vi "BIMS_Assembler.vi"() -> ()   [LabVIEW 2010]
doc: "This program is currently beta software. It is designed to address the data requirements defined primarily by the DHB Ballistic Test Report.\n\nThe general operation of this program is based on the Ballistics Version 2005 application developed internally by DuPont as a research tool for the Spruance Plant Ballistics Lab in Richmond, VA.\n\nPlease note that the original trigger control logic was modified and no longer depends on a safety interlock system to enable operation of a ballistic test.\n\nDuPont makes no warranties and assumes no liabilities in connection with any use of this program."
uses:
  Collector State.ctl
  <vilib>/registry/registry.llb/Registry RtKey.ctl
  BIMS_Collector Globals.vi
panel:
  out "Loading":u16(ring)
  in  "runtimeMenusVisible":bool=TRUE
  in  "diagPageVisible":bool
  in  "RESET All":bool
  out "ConfigName":string
  out "TimeNow":string
  in  "EXIT":bool
  in  "mainTabCntrl":enum32{"Setup", "System"}(tab)
  in  "Sample SubTabCntrl":T1(tab)
  in  "NewProject":bool
  in  "# of Panels":dbl
  in  "SampleID":string caption="Sample ID"
  in  "SampleDimensions":u16(ring) caption="Dimensions" items=["", "15 x 15", "12 x 12", "10.25 x 11.75", "15 x 16", "26 x 26", "8.5 x 11", "12 x 15", "16 x 16", "18 x 18", "20 x 16", "15 x 18", "24 x 24", "13 x 13", "7.5 x 7.5", "VEST PANEL", "CHEST PLATE", "HELMET", "NOT APPLICABLE"]
  in  "ModelMfrs":u16(ring) caption="Manufacturer" items=["DuPont Experimental", "Clark Schwebel", "Industriales Textiles", "Maydown", "Second Chance Body Armor", "Point Blank-Marine Interceptor", "Safari Land", "American Body Armor", "Europe", "Force One", "Textile Filter", "Hexcel Schwebel", "BGF", "M.C. GILL", "COLUMBIA", "Britax HEATH TECN", "ARLON", "TEX TECH INC.", "TELAIR", "CADDIN BODY ARMOR", "GEPCO", "3 TEX", "PACA BODY ARMOR", "VON ROL ISOLA", "SIOUX MANUFACTURING", "APEJ-TAIWAN", "FLOPPY BODY ARMOR", "UNICOR", "n/a", "Point Blank", "Diamond Back", "Other"]
  in  "SampleTypes":u16(ring) caption="Sample Type" items=["", "Fabric", "Hard", "Helmet", "Vest", "Paper"]
  in  "Submitters":u16(ring) caption="Submitter" items=["", "Aldo Tavarez", "James Singletary", "Jeff Hanks", "Karl Chang", "Minshon Chiou", "Other", "Navin Tejani", "Pat Fitzgerald", "Ron Egres", "Bryce VanArsdalen", "Kevin Mulcahy"]
  out "ProjectID":string caption="Project ID"
  in  "BackLayers":i32 caption="# of Layers" min=0 max=99 step=5
  in  "FrontLayers":i32 caption="# of Layers" min=0 max=99 step=5
  in  "BackLayer":u16(ring) caption="Back Layer" items=["", "n/a", "CORDURA 500d"]
  in  "FrontLayer":u16(ring) caption="Front Layer" items=["", "n/a", "CORDURA 1000d"]
  out "totalNumLayers":i32 caption="Total # of Layers" min=0 max=100 step=5
  out "totalBAW":sgl caption="Total BAW (psf)" format="%.2f"
  in  "LayerTabControl":enum32{"1", "2", "3", "4", "5", "6"}(tab) caption="Inner Layers"
  out "fab1_totalWt":sgl caption="Fab1 Wt" min=0 max=99 step=5 format="%.2f"
  out "SampleAttribs_1":T2 caption="fabricAttribs_1"
  in  "Layer_1":T3={"plyNum"=0, "LotNum"="n/a", "RollNum"="n/a"} caption="Fabric #1" {"plyNum" min=0 max=99 step=5}
  in  "SampleStyle_1":u16(ring)
  in  "Mfr_1":u16(ring) caption="vendor" items=["", "Barrday", "DSM", "DuPont AFS", "Dyneema", "Honeywell", "JPS", "TexTech"]
  in  "layerStitch_1":u16(ring) caption="Stitch" items=["", "1-inch quilt", "2-inch quilt", "Corner Bartack", "Corners", "Custom (Panel)", "Custom (Vest)", "Diamond", "Edge", "n/a", "Normal"]
  out "fab2_totalWt":sgl caption="Fab2 Wt" min=0 max=99 step=5 format="%.2f"
  out "SampleAttribs_2":T2 caption="fabricAttribs_2"
  in  "Layer_2":T3={"plyNum"=0, "LotNum"="n/a", "RollNum"="n/a"} caption="Fabric #2" {"plyNum" min=0 max=99 step=5}
  in  "SampleStyle_2":u16(ring)
  in  "Mfr_2":u16(ring) caption="vendor" items=["", "Barrday", "DSM", "DuPont AFS", "Dyneema", "Honeywell", "JPS", "TexTech"]
  in  "layerStitch_2":u16(ring) caption="Stitch" items=["", "1-inch quilt", "2-inch quilt", "Corner Bartack", "Corners", "Custom (Panel)", "Custom (Vest)", "Diamond", "Edge", "n/a", "Normal"]
  out "fab3_totalWt":sgl caption="Fab3 Wt" min=0 max=99 step=5 format="%.2f"
  out "SampleAttribs_3":T2 caption="fabricAttribs_3"
  in  "Layer_3":T3={"plyNum"=0, "LotNum"="n/a", "RollNum"="n/a"} caption="Fabric #3" {"plyNum" min=0 max=99 step=5}
  in  "SampleStyle_3":u16(ring)
  in  "Mfr_3":u16(ring) caption="vendor" items=["", "Barrday", "DSM", "DuPont AFS", "Dyneema", "Honeywell", "JPS", "TexTech"]
  in  "layerStitch_3":u16(ring) caption="Stitch" items=["", "1-inch quilt", "2-inch quilt", "Corner Bartack", "Corners", "Custom (Panel)", "Custom (Vest)", "Diamond", "Edge", "n/a", "Normal"]
  out "fab4_totalWt":sgl caption="Fab4 Wt" min=0 max=99 step=5 format="%.2f"
  out "SampleAttribs_4":T2 caption="fabricAttribs_4"
  in  "Layer_4":T3={"plyNum"=0, "LotNum"="n/a", "RollNum"="n/a"} caption="Fabric #4" {"plyNum" min=0 max=99 step=5}
  in  "SampleStyle_4":u16(ring)
  in  "Mfr_4":u16(ring) caption="vendor" items=["", "Barrday", "DSM", "DuPont AFS", "Dyneema", "Honeywell", "JPS", "TexTech"]
  in  "layerStitch_4":u16(ring) caption="Stitch" items=["", "1-inch quilt", "2-inch quilt", "Corner Bartack", "Corners", "Custom (Panel)", "Custom (Vest)", "Diamond", "Edge", "n/a", "Normal"]
  out "fab5_totalWt":sgl caption="Fab5 Wt" min=0 max=99 step=5 format="%.2f"
  out "SampleAttribs_5":T2 caption="fabricAttribs_5"
  in  "Layer_5":T3={"plyNum"=0, "LotNum"="n/a", "RollNum"="n/a"} caption="Fabric #5" {"plyNum" min=0 max=99 step=5}
  in  "SampleStyle_5":u16(ring)
  in  "Mfr_5":u16(ring) caption="vendor" items=["", "Barrday", "DSM", "DuPont AFS", "Dyneema", "Honeywell", "JPS", "TexTech"]
  in  "layerStitch_5":u16(ring) caption="Stitch" items=["", "1-inch quilt", "2-inch quilt", "Corner Bartack", "Corners", "Custom (Panel)", "Custom (Vest)", "Diamond", "Edge", "n/a", "Normal"]
  out "fab6_totalWt":sgl caption="Fab6 Wt" min=0 max=99 step=5 format="%.2f"
  out "SampleAttribs_6":T2 caption="fabricAttribs_6"
  in  "Layer_6":T3={"plyNum"=0, "LotNum"="n/a", "RollNum"="n/a"} caption="Fabric #6" {"plyNum" min=0 max=99 step=5}
  in  "SampleStyle_6":u16(ring)
  in  "Mfr_6":u16(ring) caption="vendor" items=["", "Barrday", "DSM", "DuPont AFS", "Dyneema", "Honeywell", "JPS", "TexTech"]
  in  "layerStitch_6":u16(ring) caption="Stitch" items=["", "1-inch quilt", "2-inch quilt", "Corner Bartack", "Corners", "Custom (Panel)", "Custom (Vest)", "Diamond", "Edge", "n/a", "Normal"]
  in  "SampleCoverings":u16(ring) caption="Sample Covering" items=["None", "RipStop", "Plastic bag", "Other"]
  in  "Assemblers":u16(ring) caption="Technician" items=["", "Not Known", "none", "Ron Egres", "Bryce VanArsdalen", "Mary Revels", "Matthew Street", "Patty Whitlow", "Tom Boyer"]
  in  "Thickness":dbl caption="Thickness (in)" format="%.3f"
  in  "totalSampleWt":sgl caption="Total Weight (lbs)" format="%.3f"
  in  "Comments":string caption="Remarks (optional):"
  in  "TestConditions":u16(ring) caption="Sample Condition" items=["", "Dry", "Wet", "Hot 160 DEG. F", "Cold", "Weapon Lubricant", "Motor Oil", "Conditioned", "Accelerated Aging"]
  in  "aboutTabCntrl":enum32{"About ", "Internal Use"}(tab)
  in  "RefreshMetadata":bool
  in  "PublishNewRecords":bool
  in  "clearErrors":bool
  in  "Server":string="esvrs11"
  in  "Site":string="ICE1"
  in  "processShots":bool
  in  "line direction map":i32=1792 format="%.0b"
  in  "old threat":u16
  in  "Areal Density":dbl format="%.2f"
  in  "Areal density text":string
  in  "Fabric Description":string caption="Fabric Desc"
  out "configPath":path=path "P:/Private/My Projects/AFS/BIMS/2008/BIMS_Collector.ini" caption="Configuration Path (INI)"
  in  "Threat":u16(ring) caption="Threat (long description)"
  out "massUnits":string="GRAMS" caption="Weight Units"
  out "lengthUnits":string="FOOT" caption="Distance Units"
  in  "SampleDescrip":u16(ring) caption="Misc. Sample Description (legacy)"
  in  "serialNum":string caption="Serial #"
  in  "Models":u16(ring) caption="Model #" items=["n/a"]
  out "SMErr":errorcluster
  out "U/I EvErr":errorcluster
  out "booleanDump":bool
  in  "LayerStitchTypes":u16(ring) caption="Stitch" items=["", "Custom (Vest)", "Corners", "1-inch quilt", "2-inch quilt", "Normal", "Custom (Panel)", "Corner Bartack", "Diamond", "Edge", "n/a"]
  # "Effectively restarts the application from scratch, as if the user pressed the EXIT button and then restarted the application."
  # "Configured for"
  # "Body Side"
  # "Strike Face"
  # "Layer"
  # "Mfr"
  # "Style"
  # "# of Plies"
  # "Lot"
  # "Roll"
  # "Stitch"
  # "Internal ID"
  # "Fiber"
  # "Denier"
  # "Pick"
  # "Weave"
  # "Finish"
  # "oz/yd²"
  # "Asset"
  # "Total Weight"
  # "1"
  # "2"
  # "3"
  # "4"
  # "5"
  # "6"
  # "DuPont Ballistics Information Management System\n\nBIMS\nEnterprise Edition\n\n\nSample Assembler\n\nJanuary 2009"
  # "DuET Measurement System Technologies\nDUCOM 8 695-2330 for technical support\n\nCopyright © 2009 DuPont Company"
  # "Deployment Configuration"
  # "Data items support Point Blank requirements:"
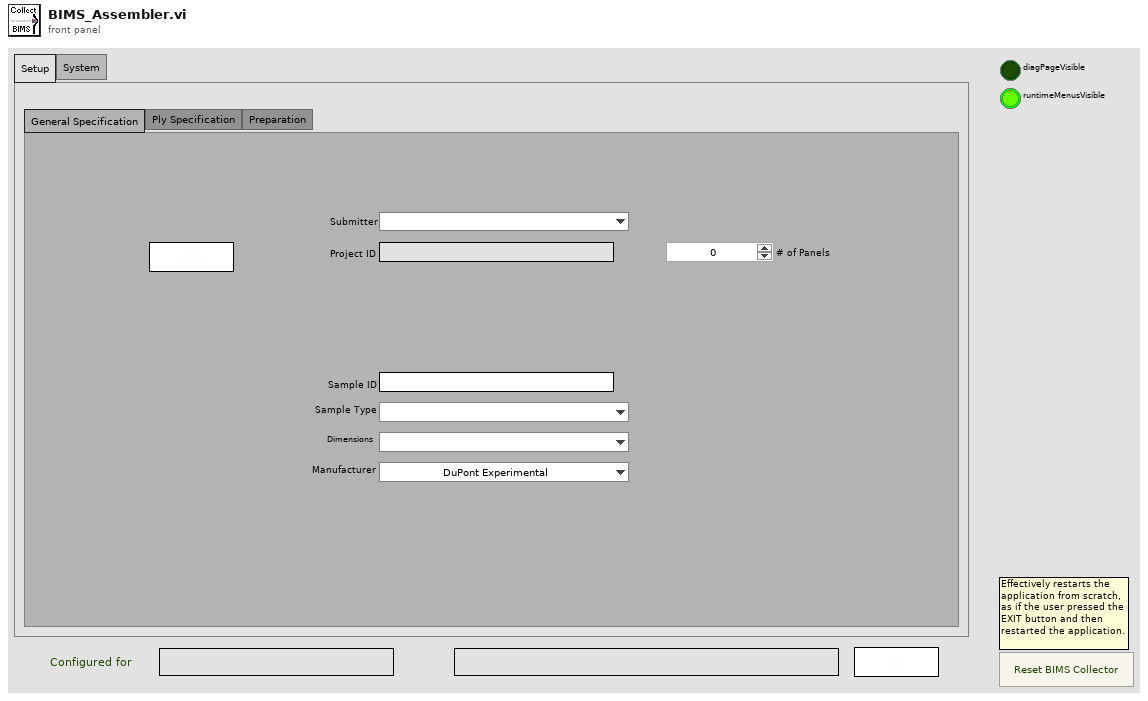
[diagram p1: front panel]
types:
  T1 = enum32{"General Specification", "Ply Specification", "Preparation"}
  T2 = cluster{"Fabric.fiber":string, "Fabric.denier":string, "pick":string, "weave":string, "finish":string, "ozPerYd2":string, "fabricID_DHB":string, "asset":string}
  T3 = cluster{"plyNum":i32, "LotNum":string, "RollNum":string}
  T4 = typedef "Collector State.ctl" = enum16{"POLL", "INITIALIZE", "V50 Report or GET Record", "VsVr Report", "SAVE SHOTS", "ADD SHOT", "CLEAR SHOTS", "NEXT SHOT", "DELETE SHOT", "PROCESS SHOTS", "READY CLOCK", "CHECK DAQ"}
  T5 = enum32{"Page Enabled", "Page Disabled", "Page Disabled & Grayed"}
  T6 = typedef "Registry RtKey.ctl" = enum32{"HKEY_CLASSES_ROOT", "HKEY_CURRENT_USER", "HKEY_LOCAL_MACHINE", "HKEY_USERS", "HKEY_PERFORMANCE_DATA", "HKEY_CURRENT_CONFIG", "HKEY_DYN_DATA"}
  T7 = cluster{"SampleTypes":refnum<vi>, "SampleDescrip":refnum<vi>}
  T8 = enum32{"invalid app kind", "Development System", "Run Time System", "Student Edition", "Embedded LabVIEW", "Evaluation", "Custom"}
  T9 = cluster{"fiber":string, "denier":string, "construction":string, "weave":string, "finish":string, "ozPerYd2":string, "fabricStyle_DHB":string, "yarnMerge":string}
  T10 = cluster{"fiber":string, "denier":string, "pick":string, "weave":string, "finish":string, "ozPerYd2":string, "internal_ID":string, "asset":string}[]
  T11 = cluster{"plyNum":i32, "LotNum":string, "RollNum":string}[]
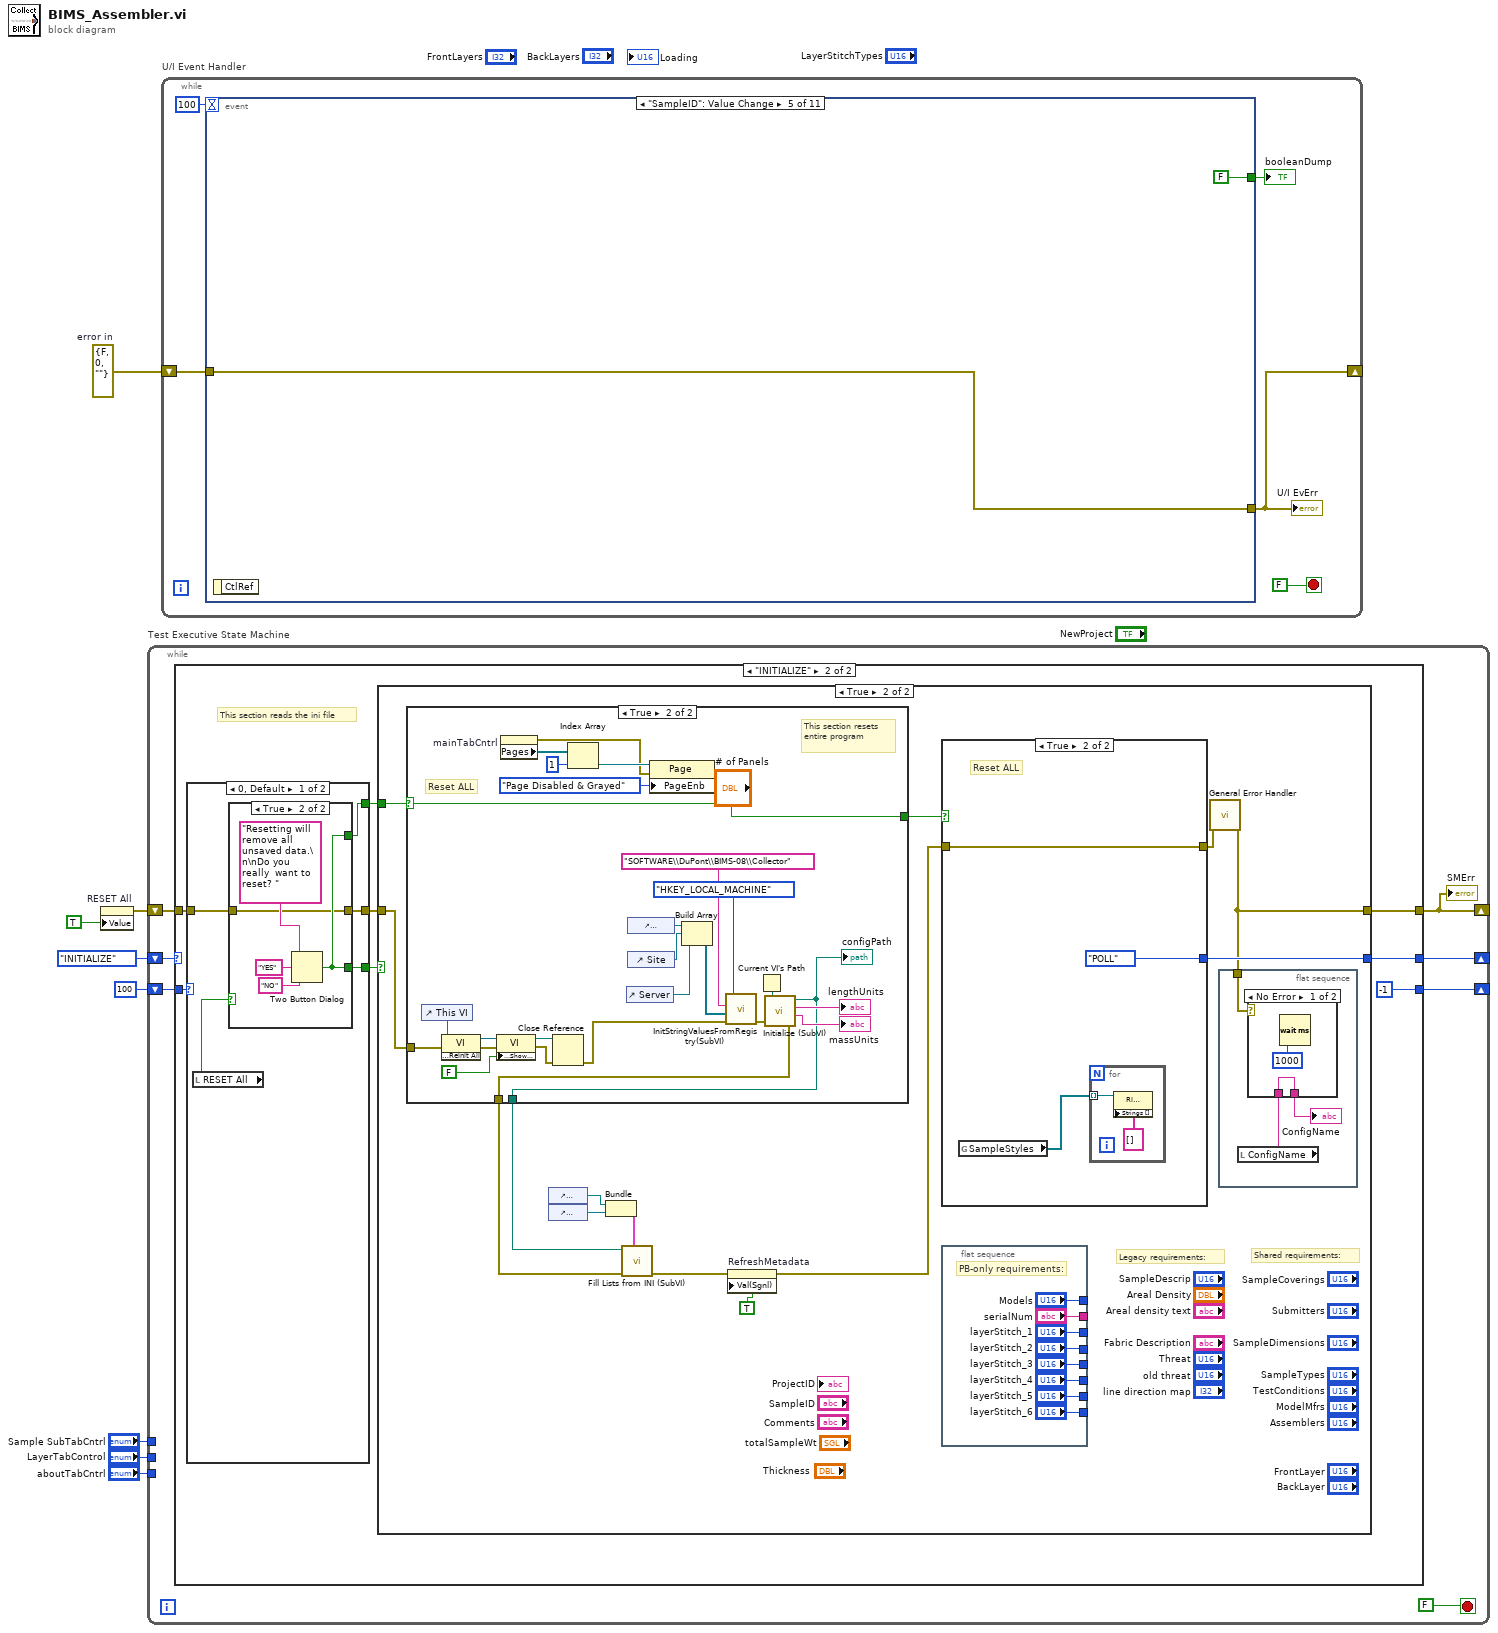
[diagram p0: block diagram]
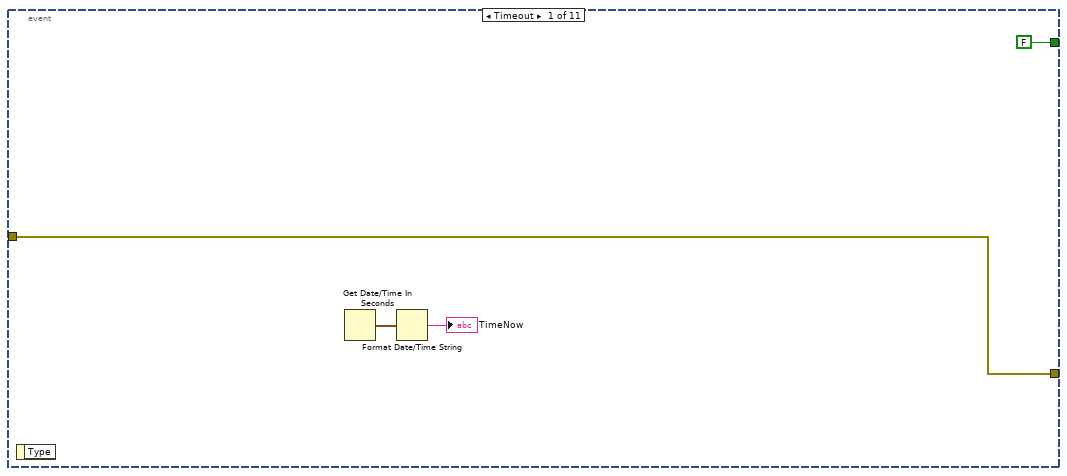
[diagram p2: hidden frame]
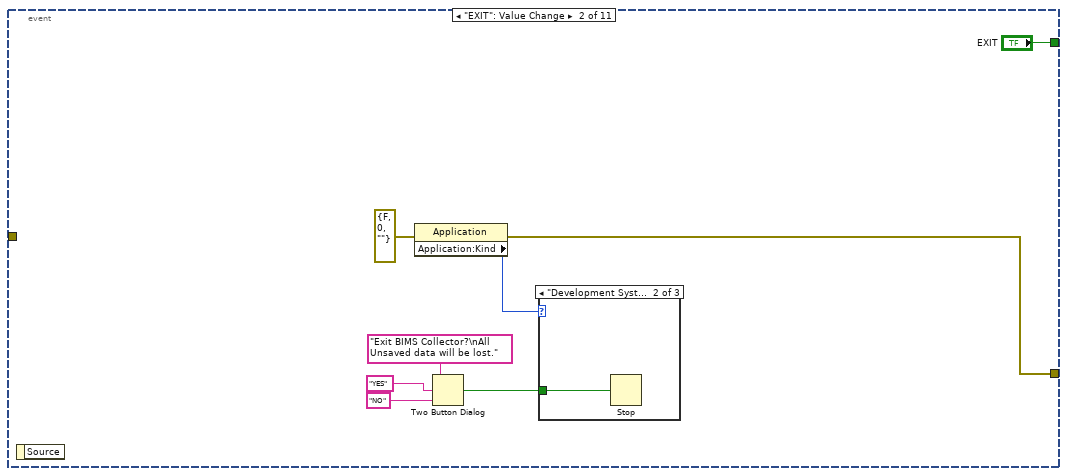
[diagram p3: hidden frame]
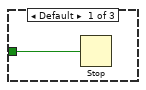
[diagram p4: hidden frame]
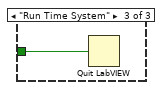
[diagram p5: hidden frame]
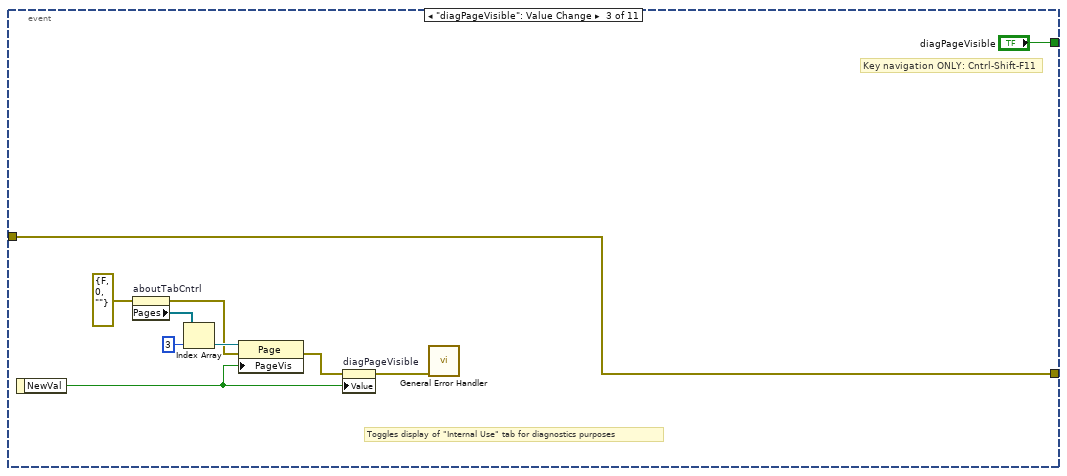
[diagram p6: hidden frame]
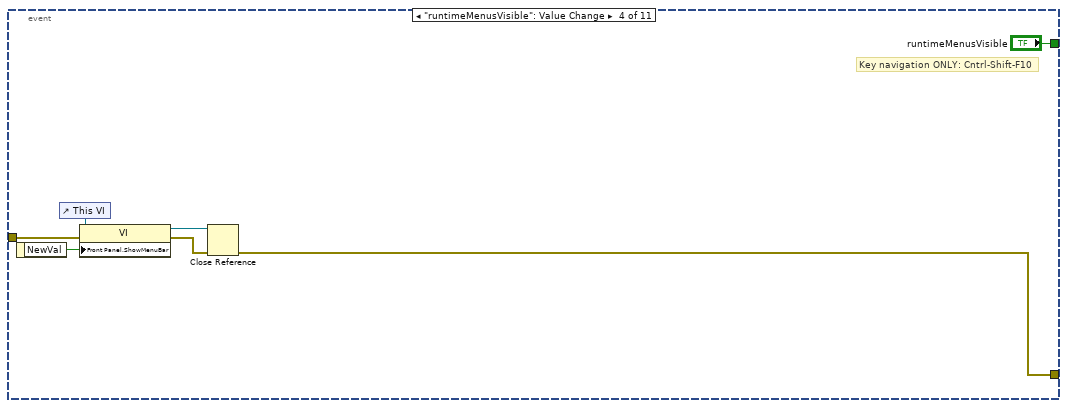
[diagram p7: hidden frame]
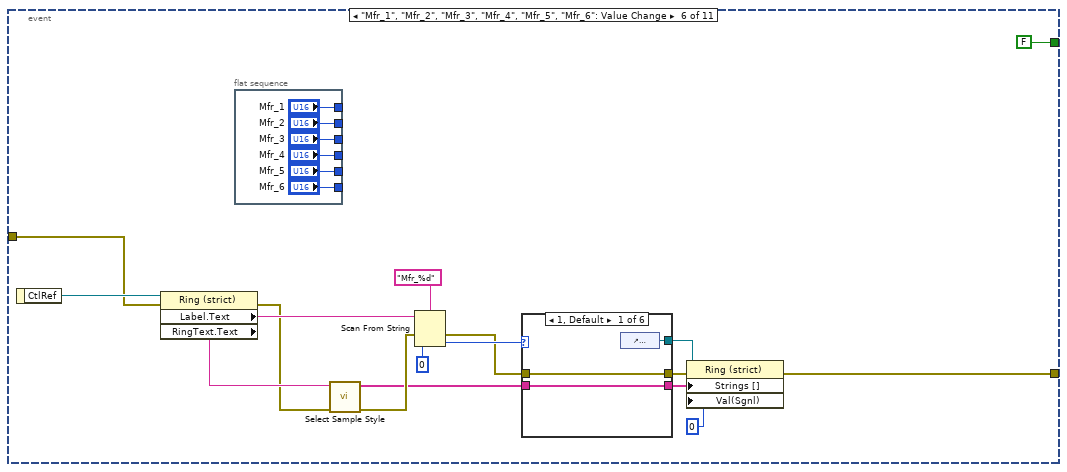
[diagram p8: hidden frame]
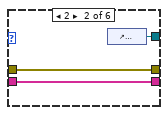
[diagram p9: hidden frame]
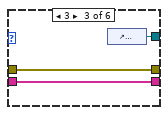
[diagram p10: hidden frame]
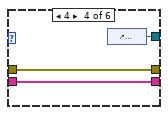
[diagram p11: hidden frame]
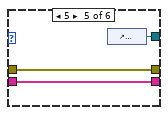
[diagram p12: hidden frame]
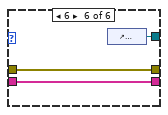
[diagram p13: hidden frame]
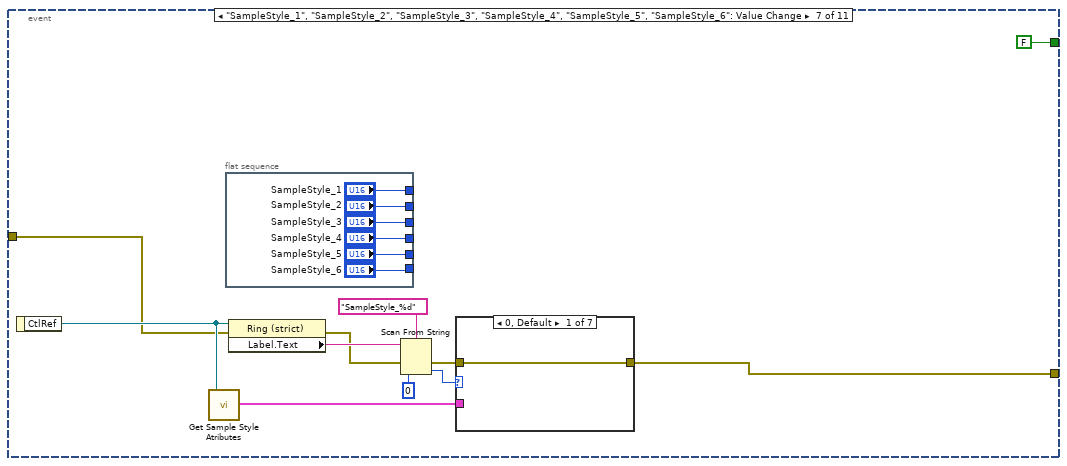
[diagram p14: hidden frame]
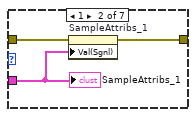
[diagram p15: hidden frame]
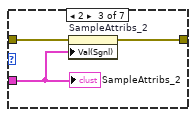
[diagram p16: hidden frame]
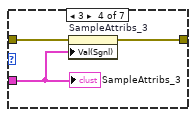
[diagram p17: hidden frame]
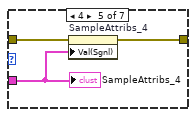
[diagram p18: hidden frame]
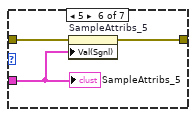
[diagram p19: hidden frame]
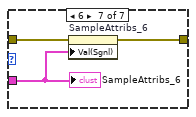
[diagram p20: hidden frame]
diagram:
  w4 = errorcluster {"status"=FALSE, "code"=0, "source"=""}  # error in
  n1 = property on="RESET All" class="Bool (strict)"("Value"=TRUE ("RESET")) -> (error out=w6:errorcluster)  [unwired: 2 in, 1 out]
  n2 = while "Test Executive State Machine" {
    shift-left: 100 -> [w12]
    shift-right: [w13] -> _
    shift-left: Collector_State."INITIALIZE" ("progState") -> [w11]
    shift-right: [w14] -> _
    shift-right: [w9] -> _
    shift-left: w6 -> [w10]
    tunnel: "LayerTabControl" -> [_]
    tunnel: "aboutTabCntrl" -> [_]
    tunnel: "Sample SubTabCntrl" -> [_]
    stop <- FALSE stop-if-true
    n3 = case shown="\"INITIALIZE\"" w11 {
      tunnel: [w22 w33] -> w14
      tunnel: [-1 -1 ("index of element")] -> w13
      tunnel: w12 -> [_ w34]
      tunnel: w10 -> [_ w29]
      tunnel: [w17 w30] -> w9
      frame "POLL", Default {
        w26 = Collector_State."POLL"  # progStateType
        w23 = TRUE  # element
        # "This section checks for any buttons, maintains routine check of the paramters"
        n4 = Build Array("RESET All", "processShots") -> (w24:bool[])
        n5 = Search 1D Array(1D array=w24, element=w23) -> (index of element=w27:i32)  [unwired: 1 out]
        n6 = Increment(x=w27) -> (x+1=w16:i32)
        n7 = local read "SMErr"() -> (w17:errorcluster)
        n8 = To Variant(anything=w16) -> (Variant=w25:variant)
        n9 = Variant To Data(Variant=w25, type=w26) -> (data=w22:T4)  [unwired: 1 in, 1 out]
        n10 = Wait (ms)(milliseconds to wait=u32 200 ("millisecond timer value")) -> ()  [unwired: 1 out]
      }
      frame "INITIALIZE" {
        # "This section reads the ini file"
        n11 = case shown="0, Default" w34 {
          tunnel: [w40 w58] -> w35
          tunnel: [w38 w58] -> w32
          tunnel: w29 -> [w37 w50]
          tunnel: [w36 w50] -> w28
          frame 0, Default {
            n12 = local read "RESET All"() -> (w39:bool)
            n13 = case shown="True" w39 {
              tunnel: [TRUE w47] -> w40
              tunnel: [FALSE w47] -> w38
              tunnel: w37 -> [w41 w44]
              tunnel: [w41 w44] -> w36
              frame False {
                # "Refresh"
              }
              frame True {
                n14 = Two Button Dialog(message="Resetting will remove all unsaved data.\n\nDo you really  want to reset? ", 1:"NO" ("F button name (\"Cancel\")"), 2:"YES" ("T button name (\"OK\")")) -> (T button?=w47:bool)
              }
            }
          }
          frame 100 {
            w58 = TRUE  # Reset ALL
            n15 = property on="Loading" class="Ring (strict)"("Visible"=FALSE) -> ()  [unwired: 2 in, 2 out]
            n16 = control-ref of="Mfr_1"() -> (w57:refnum<vi>)
            n17 = control-ref of="Mfr_2"() -> (w56:refnum<vi>)
            n18 = control-ref of="Mfr_3"() -> (w55:refnum<vi>)
            n19 = control-ref of="Mfr_4"() -> (w54:refnum<vi>)
            n20 = control-ref of="Mfr_5"() -> (w53:refnum<vi>)
            n21 = control-ref of="Mfr_6"() -> (w52:refnum<vi>)
            n22 = Build Array(w57, w56, w55, w54, w53, w52) -> (w51:refnum<vi>[])
            n23 = global write "BIMS_Collector Globals.vi" "Mfrs"(w51) -> ()
          }
        }
        n24 = case shown="True" w35 {
          tunnel: [Collector_State."POLL" ("progState") w74] -> w33
          tunnel: w32 -> [_ w75]
          tunnel: [w59 w66] -> w30
          tunnel: w28 -> [w59 w73]
          frame False {
            n25 = local write "RESET All"(FALSE ("RESET")) -> ()
          }
          frame True {
            # "Legacy requirements:"
            # "Shared requirements:"
            n26 = case shown="True" w75 {
              selector: w75 -> [_ w106]
              tunnel: [w92 w106] -> w67
              tunnel: [w91 w115] -> w63
              tunnel: w73 -> [w91 w108]
              tunnel: [w90 w105] -> w64
              frame False {
                w92 = FALSE  # Reset All
                # "Refresh"
                n27 = local read "configPath"() -> (w90:path)
              }
              frame True {
                # "This section resets\nentire program"
                # "Reset ALL"
                n28 = control-ref of="This VI"() -> (w99:refnum<vi>)
                n29 = invoke on="Invoke Node" class="VI" method="Default Vals.Reinit All"(reference=w99, error in=w108) -> (reference out=w98:refnum<vi>, error out=w97:errorcluster)  [unwired: 1 in, 1 out]
                n30 = property class="VI"(reference=w98, error in=w97, "Front Panel.ShowMenuBar"=FALSE ("Front Panel Window:Show Menu Bar")) -> (reference out=w95:refnum<vi>, error out=w94:errorcluster)
                n31 = property on="mainTabCntrl" class="TabCtl (strict)"() -> (error out=w100:errorcluster, "Pages"=w102:refnum<vi>[])  [unwired: 2 in, 1 out]
                n32 = Close Reference(reference=w95, error in (no error)=w94) -> (error out=w93:errorcluster)
                n33 = Index Array(array=w102, index=1) -> (element=w104:refnum<vi>)
                n34 = control-ref of="Server"() -> (w107:refnum<vi>)
                n35 = control-ref of="ConfigName"() -> (w111:refnum<vi>)
                n36 = control-ref of="Site"() -> (w109:refnum<vi>)
                n37 = property on="Property Node" class="Page"(reference=w104, error in=w100, "PageEnb"=T5."Page Disabled & Grayed" ("Page Enabled State")) -> ()  [unwired: 2 out]
                n38 = Build Array(w111, w109, w107) -> (w112:refnum<vi>[])
                n39 = call "InitStringValuesFromRegistry(SubVI).vi"("error in"=w93, "String References"=w112, "subkey"="SOFTWARE\\DuPont\\BIMS-08\\Collector", "root key (HKEY_LOCAL_MACHINE)"=Registry_RtKey."HKEY_LOCAL_MACHINE") -> ("error out"=w114:errorcluster)  [unwired: 3 out]
                n40 = Current VI's Path() -> (path=w118:path)
                n41 = call "Initialize (SubVI).vi"("path"=w118, "error IN"=w114) -> ("pathConfigOUT"=w105:path, "lengthUnits"=→"lengthUnits":string, "massUnits"=→"massUnits":string, "error out"=w115:errorcluster)  [unwired: 1 out]
                "configPath" <- w105
              }
            }
            n42 = control-ref of="SampleTypes"() -> (w69:refnum<vi>)
            n43 = control-ref of="SampleDescrip"() -> (w71:refnum<vi>)
            n44 = Bundle("SampleTypes"=w69, "SampleDescrip"=w71) -> (w70:T7)  [unwired: 1 out]
            n45 = call "Fill Lists from INI (SubVI).vi"("clusterListboxes"=w70, "error in"=w63, "pathConfigIN"=w64) -> ("error out"=w62:errorcluster)  [unwired: 5 out]
            n46 = property on="RefreshMetadata" class="Bool (strict)"(error in=w62, "Val(Sgnl)"=TRUE) -> (error out=w65:errorcluster)  [unwired: 1 in, 1 out]
            n47 = case shown="True" w67 {
              tunnel: [Collector_State."POLL" ("progState") Collector_State."POLL" ("progState")] -> w74
              tunnel: [w119 w121] -> w72
              tunnel: w65 -> [w119 w121]
              frame False {
                # "Refresh"
              }
              frame True {
                # "Reset ALL"
                n48 = global read "BIMS_Collector Globals.vi" "SampleStyles"() -> (w122:refnum<vi>[])
                n49 = for {
                  tunnel: w122 -> [w124] mode=indexing
                  n50 = property on="Property Node" class="Ring (strict)"(reference=w124, "Strings []"=string[] []) -> ()  [unwired: 1 in, 2 out]
                }
              }
            }
            n51 = flat-sequence {
              tunnel: ["Models"] -> _
              tunnel: ["serialNum"] -> _
              tunnel: ["layerStitch_1"] -> _
              tunnel: ["layerStitch_2"] -> _
              tunnel: ["layerStitch_3"] -> _
              tunnel: ["layerStitch_4"] -> _
              tunnel: ["layerStitch_5"] -> _
              tunnel: ["layerStitch_6"] -> _
              frame #0 {
                # "PB-only requirements:"
              }
            }
            n52 = call <vilib>:"General Error Handler.vi"("error in (no error)"=w72) -> ("error out"=w66:errorcluster)  [unwired: 1 in, 13 out]
            n53 = flat-sequence {
              tunnel: w66 -> [w84]
              frame #0 {
                n54 = local read "ConfigName"() -> (w85:string)
                n55 = case shown="No Error" w84 {
                  tunnel: [w88 "NOT READY!" ("ConfigName")] -> w86
                  tunnel: w85 -> [w88 _]
                  frame No Error {
                    n56 = Wait (ms)(milliseconds to wait=u32 1000) -> ()  [unwired: 1 out]
                  }
                  frame Error {
                  }
                }
                "ConfigName" <- w86
              }
            }
          }
        }
      }
    }
    "SMErr" <- w9
  }
  n57 = while "U/I Event Handler" {
    shift-right: [w127] -> _
    shift-left: w4 -> [w128]
    stop <- FALSE stop-if-true
    n58 = event shown="[4] \"SampleID\": Value Change" {
      selector: _ -> [_ _ _ _ _ _ _ _ _ _ _]
      dyn-events: _ -> [_ _ _ _ _ _ _ _ _ _ _]
      timeout: 100 -> [_ _ _ _ _ _ _ _ _ _ _]
      tunnel: w128 -> [w132 _ w149 w159 w163 w173 w210 w243 w284 w320 _]
      tunnel: [w132 w136 w149 w156 w163 w172 w207 w243 w281 w322 w343] -> w127
      tunnel: [FALSE ("UpdateMetadata") "EXIT" "diagPageVisible" "runtimeMenusVisible" FALSE ("UpdateMetadata") FALSE ("UpdateMetadata") FALSE ("UpdateMetadata") FALSE ("UpdateMetadata") "PublishNewRecords" "RefreshMetadata" FALSE ("UpdateMetadata")] -> w126
      event Timeout {
        n59 = event-data() -> ()  [unwired: 2 out]
        n60 = Get Date/Time In Seconds() -> (seconds since 1Jan1904=w134:timestamp)
        n61 = Format Date/Time String(seconds (now)=w134) -> (date/time string=→"TimeNow":string)  [unwired: 2 out]
      }
      event "EXIT": Value Change {
        n62 = event-data() -> ()  [unwired: 2 out]
        n63 = property on="Property Node" class="Application"(error in=errorcluster {"status"=FALSE, "code"=0, "source"=""} ("error in (no error)")) -> (error out=w136:errorcluster, "Application:Kind"=w141:T8)  [unwired: 1 in, 1 out]
        n64 = Two Button Dialog(message="Exit BIMS Collector?\nAll Unsaved data will be lost.", 1:"NO" ("F button name (\"Cancel\")"), 2:"YES" ("T button name (\"OK\")")) -> (T button?=w142:bool)
        n65 = case shown="\"Development System\"" w141 {
          tunnel: w142 -> [w143 w144 w145]
          frame Default {
            n66 = Stop(stop? (T)=w143) -> ()
          }
          frame "Development System" {
            n67 = Stop(stop? (T)=w144) -> ()
          }
          frame "Run Time System" {
            n68 = Quit LabVIEW(quit? (T)=w145) -> ()
          }
        }
      }
      event "diagPageVisible": Value Change {
        # "Toggles display of \"Internal Use\" tab for diagnostics purposes"
        # "Key navigation ONLY: Cntrl-Shift-F11"
        n69 = event-data() -> ("NewVal"=w152:bool)  [unwired: 1 out]
        n70 = property on="aboutTabCntrl" class="TabCtl (strict)"(error in=errorcluster {"status"=FALSE, "code"=0, "source"=""} ("error in (no error)")) -> (error out=w151:errorcluster, "Pages"=w155:refnum<vi>[])  [unwired: 1 in, 1 out]
        n71 = Index Array(array=w155, index=3) -> (element=w153:refnum<vi>)
        n72 = property on="Property Node" class="Page"(reference=w153, error in=w151, "PageVis"=w152) -> (error out=w150:errorcluster)  [unwired: 1 out]
        n73 = property on="diagPageVisible" class="Bool (strict)"(error in=w150, "Value"=w152) -> (error out=w147:errorcluster)  [unwired: 1 in, 1 out]
        n74 = call <vilib>:"General Error Handler.vi"("error in (no error)"=w147) -> ()  [unwired: 1 in, 14 out]
      }
      event "runtimeMenusVisible": Value Change {
        # "Key navigation ONLY: Cntrl-Shift-F10"
        n75 = event-data() -> ("NewVal"=w161:bool)  [unwired: 1 out]
        n76 = control-ref of="This VI"() -> (w160:refnum<vi>)
        n77 = property class="VI"(reference=w160, error in=w159, "Front Panel.ShowMenuBar"=w161) -> (reference out=w158:refnum<vi>, error out=w157:errorcluster)
        n78 = Close Reference(reference=w158, error in (no error)=w157) -> (error out=w156:errorcluster)
      }
      event "SampleID": Value Change {
        n79 = event-data() -> ()  [unwired: 2 out]
      }
      event "Mfr_1", "Mfr_2", "Mfr_3", "Mfr_4", "Mfr_5", "Mfr_6": Value Change {
        n80 = event-data() -> ("CtlRef"=w181:refnum<vi>)  [unwired: 1 out]
        n81 = property on="Property Node" class="Ring (strict)"(reference=w181, error in=w173) -> (error out=w171:errorcluster, "Label.Text"=w177:string, "RingText.Text"=w178:string)  [unwired: 1 out]
        n82 = flat-sequence {
          tunnel: ["Mfr_1"] -> _
          tunnel: ["Mfr_2"] -> _
          tunnel: ["Mfr_3"] -> _
          tunnel: ["Mfr_4"] -> _
          tunnel: ["Mfr_5"] -> _
          tunnel: ["Mfr_6"] -> _
          frame #0 {
          }
        }
        n83 = call "Select Sample Style.vi"("error IN"=w171, "Mfr"=w178) -> ("error Out"=w170:errorcluster, "SampleStyles"=w166:string[])  [unwired: 4 out]
        n84 = Scan From String(format string="Mfr_%d", input string=w177, error in=w170, default 1=0 ("Mfr#")) -> (error out=w167:errorcluster, output 1=w176:i32)  [unwired: 1 in, 2 out]
        n85 = case shown="1, Default" w176 {
          tunnel: [w190 w193 w196 w199 w202 w205] -> w175
          tunnel: [w189 w192 w195 w198 w201 w204] -> w168
          tunnel: w167 -> [w189 w192 w195 w198 w201 w204]
          tunnel: w166 -> [w188 w191 w194 w197 w200 w203]
          tunnel: [w188 w191 w194 w197 w200 w203] -> w165
          frame 1, Default {
            n86 = control-ref of="SampleStyle_1"() -> (w190:refnum<vi>)
          }
          frame 2 {
            n87 = control-ref of="SampleStyle_2"() -> (w193:refnum<vi>)
          }
          frame 3 {
            n88 = control-ref of="SampleStyle_3"() -> (w196:refnum<vi>)
          }
          frame 4 {
            n89 = control-ref of="SampleStyle_4"() -> (w199:refnum<vi>)
          }
          frame 5 {
            n90 = control-ref of="SampleStyle_5"() -> (w202:refnum<vi>)
          }
          frame 6 {
            n91 = control-ref of="SampleStyle_6"() -> (w205:refnum<vi>)
          }
        }
        n92 = property on="Property Node" class="Ring (strict)"(reference=w175, error in=w168, "Strings []"=w165, "Val(Sgnl)"=u16 0 ("Value (Signaling)")) -> (error out=w172:errorcluster)  [unwired: 1 out]
      }
      event "SampleStyle_1", "SampleStyle_2", "SampleStyle_3", "SampleStyle_4", "SampleStyle_5", "SampleStyle_6": Value Change {
        n93 = event-data() -> ("CtlRef"=w216:refnum<vi>)  [unwired: 1 out]
        n94 = call "Get Sample Style Atributes.vi"("StyleNumRef"=w216) -> ("SampleSpecs"=w211:T9)  [unwired: 1 in]
        n95 = flat-sequence {
          tunnel: ["SampleStyle_1"] -> _
          tunnel: ["SampleStyle_2"] -> _
          tunnel: ["SampleStyle_3"] -> _
          tunnel: ["SampleStyle_4"] -> _
          tunnel: ["SampleStyle_5"] -> _
          tunnel: ["SampleStyle_6"] -> _
          frame #0 {
          }
        }
        n96 = property on="Property Node" class="Ring (strict)"(reference=w216, error in=w210) -> (error out=w209:errorcluster, "Label.Text"=w215:string)  [unwired: 1 out]
        n97 = Scan From String(format string="SampleStyle_%d", input string=w215, error in=w209, default 1=0 ("default value 1")) -> (error out=w208:errorcluster, output 1=w213:i32)  [unwired: 1 in, 2 out]
        n98 = case shown="0, Default" w213 {
          tunnel: w211 -> [_ w226 w229 w232 w235 w238 w241]
          tunnel: w208 -> [w223 w225 w228 w231 w234 w237 w240]
          tunnel: [w223 w224 w227 w230 w233 w236 w239] -> w207
          frame 0, Default {
          }
          frame 1 {
            n99 = property on="SampleAttribs_1" class="Clust (strict)"(error in=w225, "Val(Sgnl)"=w226) -> (error out=w224:errorcluster)  [unwired: 1 in, 1 out]
            "SampleAttribs_1" <- w226
          }
          frame 2 {
            n100 = property on="SampleAttribs_2" class="Clust (strict)"(error in=w228, "Val(Sgnl)"=w229) -> (error out=w227:errorcluster)  [unwired: 1 in, 1 out]
            "SampleAttribs_2" <- w229
          }
          frame 3 {
            n101 = property on="SampleAttribs_3" class="Clust (strict)"(error in=w231, "Val(Sgnl)"=w232) -> (error out=w230:errorcluster)  [unwired: 1 in, 1 out]
            "SampleAttribs_3" <- w232
          }
          frame 4 {
            n102 = property on="SampleAttribs_4" class="Clust (strict)"(error in=w234, "Val(Sgnl)"=w235) -> (error out=w233:errorcluster)  [unwired: 1 in, 1 out]
            "SampleAttribs_4" <- w235
          }
          frame 5 {
            n103 = property on="SampleAttribs_5" class="Clust (strict)"(error in=w237, "Val(Sgnl)"=w238) -> (error out=w236:errorcluster)  [unwired: 1 in, 1 out]
            "SampleAttribs_5" <- w238
          }
          frame 6 {
            n104 = property on="SampleAttribs_6" class="Clust (strict)"(error in=w240, "Val(Sgnl)"=w241) -> (error out=w239:errorcluster)  [unwired: 1 in, 1 out]
            "SampleAttribs_6" <- w241
          }
        }
      }
      event "Layer_1.plyNum", "Layer_2.plyNum", "Layer_3.plyNum", "Layer_4.plyNum", "Layer_5.plyNum", "Layer_6.plyNum", "SampleAttribs_1.ozPerYd2", "SampleAttribs_2.ozPerYd2", "SampleAttribs_3.ozPerYd2", "SampleAttribs_4.ozPerYd2", "SampleAttribs_5.ozPerYd2", "SampleAttribs_6.ozPerYd2": Value Change {
        n105 = event-data() -> ()  [unwired: 2 out]
        n106 = global read "BIMS_Collector Globals.vi" "SampleAttribs"() -> (w251:T10)
        n107 = Build Array("Layer_1", "Layer_2", "Layer_3", "Layer_4", "Layer_5", "Layer_6") -> (w244:T11)
        n108 = global write "BIMS_Collector Globals.vi" "LayerSpecs"(w244) -> ()
        n109 = for {
          tunnel: w244 -> [w272] mode=indexing
          shift-right: [w274] -> w253
          shift-left: 0 -> [w273]
          tunnel: [w271] -> w263 mode=indexing
          tunnel: w251 -> [w269] mode=indexing
          n110 = Unbundle By Name(w269) -> ("ozPerYd2"=w265:string)
          n111 = Equal?(x=w265, y="" ("Empty String Constant")) -> (x = y?=w264:bool)
          n112 = case shown="False" w264 {
            tunnel: [w278 sgl 0.0 ("default value 1")] -> w268
            tunnel: w265 -> [w275 _]
            frame False {
              n113 = Scan From String(format string="%f", input string=w275, default 1=sgl 0.0 ("default value 1")) -> (output 1=w278:sgl)  [unwired: 2 in, 3 out]
            }
            frame True {
            }
          }
          n114 = Unbundle By Name(w272) -> ("plyNum"=w270:i32)
          n115 = Add(x=w273, y=w270) -> (x+y=w274:i32)
          n116 = To Single Precision Float(number=w270) -> (single precision float=w267:sgl)
          n117 = Multiply(x=w267, y=w268) -> (x*y=w271:sgl)
        }
        "totalNumLayers" <- w253
        n118 = Divide(x=w263, y=sgl 144.0) -> (x/y=w261:sgl[])
        n119 = Index Array(array=w261) -> (element #1=→"fab1_totalWt":sgl, element #2=→"fab2_totalWt":sgl, element #3=→"fab3_totalWt":sgl, element #4=→"fab4_totalWt":sgl, element #5=→"fab5_totalWt":sgl, element #6=→"fab6_totalWt":sgl)  [unwired: 6 in]
        n120 = Add Array Elements(numeric array=w261) -> (sum=→"totalBAW":sgl)
      }
      event "PublishNewRecords": Value Change {
        w294 = "\\" ("string")
        w297 = TRUE  # overwrite (F)
        # "2. INSERT new records to Experiments and  \n      Shots tables in local Export.mdb file."
        # "1. SELECT new records from local MDB \n     by comparing against last record numbers \n     found in IMPORT table on BIMS server."
        # "Pushes latest ballistics performance data up to BIMS Server\n\n - Attempts connection with server (reports connection success in msgbox)\n - If successful:\n   - Exports all experiment/shot records since last table marker to [site].mdb file\n   - Sends export.mdb file to drop location on BIMS File Server\n   - Executes SSIS package to import records from export.mdb file\n - Otherwise provides option to try again or cancel"
        # "3. Copy Export.mdb file to [sitename].mdb in [sitename] \n      FileDrop folder on BIMS server."
        n121 = event-data() -> ()  [unwired: 2 out]
        n122 = property on="Loading" class="Ring (strict)"(error in=w284, "Visible"=TRUE) -> (error out=w283:errorcluster)  [unwired: 1 in, 1 out]
        n123 = local read "Site"() -> (w289:string)
        n124 = call "Export New Records.vi"("error IN"=w283, "Site"=w289) -> ("error out"=w299:errorcluster)  [unwired: 3 in, 6 out]
        n125 = Concatenate Strings("\\\\" ("string"), "Server", w294, "icela_" ("string"), "Server", "\\BIMS\\File Drops" ("string"), w294, w289, w294, w289, ".mdb" ("string")) -> (w291:string)
        n126 = String To Path(string=w291) -> (path=w287:path)
        n127 = Copy(8:w299, 9:w297, 10:w287, 11:path "C:/Ballistics/Export.mdb" ("source path")) -> (0:w296:errorcluster)  [unwired: 3 out]
        n128 = case shown="No Error" w296 {
          selector: w296 -> [w301 w303]
          tunnel: [w301 w302] -> w282
          frame No Error {
            n129 = One Button Dialog(message="New sample performance records submitted \nto BIMS Warehouse successfully.\n\nPublishing will occur in under five minutes.") -> ()  [unwired: 2 out]
          }
          frame Error {
            n130 = call <vilib>:"General Error Handler.vi"("error in (no error)"=w303) -> ("error out"=w302:errorcluster)  [unwired: 1 in, 13 out]
          }
        }
        n131 = property on="Loading" class="Ring (strict)"(error in=w282, "Visible"=FALSE) -> (error out=w281:errorcluster)  [unwired: 1 in, 1 out]
      }
      event "RefreshMetadata": Value Change {
        # "Pulls latest metadata down from BIMS Database Server\n - Attempts connection with server \n        (reports failure if connection is unsuccessful)\n - If successful:\n   - Updates local database records from server\n   - Updates dropdown listboxes from local database"
        n132 = event-data() -> ()  [unwired: 2 out]
        n133 = property on="Loading" class="Ring (strict)"(error in=w320, "Visible"=TRUE) -> (error out=w319:errorcluster)  [unwired: 1 in, 1 out]
        n134 = control-ref of="LayerStitchTypes"() -> (w304:refnum<vi>)
        n135 = control-ref of="BackLayer"() -> (w316:refnum<vi>)
        n136 = control-ref of="FrontLayer"() -> (w317:refnum<vi>)
        n137 = control-ref of="SampleTypes"() -> (w335:refnum<vi>)
        n138 = control-ref of="SampleDimensions"() -> (w334:refnum<vi>)
        n139 = control-ref of="ModelMfrs"() -> (w333:refnum<vi>)
        n140 = control-ref of="Assemblers"() -> (w332:refnum<vi>)
        n141 = control-ref of="Submitters"() -> (w331:refnum<vi>)
        n142 = control-ref of="TestConditions"() -> (w328:refnum<vi>)
        n143 = Build Array(w304, w316, w317, w335, w334, w333, w332, w331, w328) -> (w330:refnum<vi>[])
        n144 = call "Update Metadata using listbox names.vi"("error in"=w319, "Site"="Site", "RefNumArrIn"=w330) -> ("error out"=w336:errorcluster, "RefNumArrOut"=w329:refnum<vi>[])  [unwired: 7 out]
        n145 = call "Fill Lists from DB (1st Pass).vi"("error in"=w336, "RefNumArray"=w329) -> ("error out"=w306:errorcluster)  [unwired: 1 in, 4 out]
        n146 = call "Fill Stitch Lists.vi"("error IN"=w306) -> ("error OUT"=w305:errorcluster)  [unwired: 6 in]
        n147 = flat-sequence {
          frame #0 {
            n148 = local write "RefreshMetadata"(FALSE ("UpdateMetadata")) -> ()
            n149 = local write "TimeNow"("Connecting to BIMS Server . . ." ("TimeNow")) -> ()
          }
        }
        n150 = call "Create local tables from Server DB.vi"("error in"=w305, "Site"="Site", "tableNames"=string[] ["Threats", "ThreatDetails", "ThreatCalibers", "Mfrs", "SampleStyles", "SampleSpecs", "FiberTypes"]) -> ("error out"=w326:errorcluster)  [unwired: 8 out]
        n151 = call "Fill Lists From DB (3rd Pass).vi"("error IN"=w326) -> ("error OUT"=w308:errorcluster)  [unwired: 3 in, 3 out]
        n152 = control-ref of="ModelMfrs"() -> (w315:refnum<vi>)
        n153 = property class="Ring (strict)"(reference=w315, error in=w308) -> (reference out=w314:refnum<vi>, error out=w313:errorcluster, "Strings []"=w312:string[])
        n154 = Delete From Array(array=w312, length=1, index=0) -> (array with subset deleted=w311:string[])  [unwired: 1 out]
        n155 = property class="Ring (strict)"(reference=w314, error in=w313, "Strings []"=w311) -> (error out=w307:errorcluster)  [unwired: 1 out]
        n156 = case shown="No Error" w307 {
          selector: w307 -> [w337 w340]
          tunnel: [w337 w340] -> w323
          frame No Error {
            n157 = local write "TimeNow"("Collector Metadata is READY!" ("TimeNow")) -> ()
            n158 = Wait (ms)(milliseconds to wait=u32 2000) -> ()  [unwired: 1 out]
          }
          frame Error {
            n159 = call <vilib>:"General Error Handler.vi"("error in (no error)"=w340) -> ()  [unwired: 1 in, 14 out]
          }
        }
        n160 = property on="Loading" class="Ring (strict)"(error in=w323, "Visible"=FALSE) -> (error out=w322:errorcluster)  [unwired: 1 in, 1 out]
      }
      event "clearErrors": Value Change {
        w343 = errorcluster {"status"=FALSE, "code"=0, "source"=""} ("error in")
        n161 = event-data() -> ()  [unwired: 7 out]
        n162 = local write "SMErr"(w343) -> ()
      }
    }
    "U/I EvErr" <- w127
    "booleanDump" <- w126
  }
